vi "LDA_analogue_start_time_sync_PN.vi"(4 "Correlation peak fit method":enum32{"Max", "Quadratic", "Gaussian"}(ring)=enum."Quadratic", 5 "Pulse high threshold (Volts)":dbl=2.5, 6 "Analogue dt (s)":dbl, 7 "Analogue LDA burst pulse array":dbl[](array[numeric]), 8 "LDA arrival dt array":dbl[](array[numeric])) -> (1 "valid bursts checksum status":bool=TRUE, 2 "Absolute LDA times (s)":dbl[](array[numeric]), 3 "LDA start time rel. to Analogue (s)":dbl)   [LabVIEW 2010]
uses:
  <vilib>/Analysis/2dsp.llb/1D Cross Correlation (DBL).vi
  <vilib>/Analysis/1siggen.llb/Ramp Pattern by Samples.vi
  <vilib>/analysis/polynomials.llb/nth Derivative of Polynomial (DBL).vi
  <vilib>/analysis/polynomials.llb/Polynomial Roots (DBL).vi
  <vilib>/Analysis/NI_AALPro.lvlib
  <vilib>/Analysis/NI_AALBase.lvlib
panel:
  out "Xcorr LDA timings":cluster{"Ramp Pattern":dbl[], dbl[]}[](graph)
  in  "Pts. either side of peak to use in fit":i32=3
  out "Analogue LDA burst pulse array":cluster{"index (row)":dbl, dbl, "Vout":dbl[]}(graph)
  out "Thresholded LDA burst times (valid only)":cluster{"index (row)":dbl, dbl, "Vout":dbl[]}(graph)
  out "Thresholded LDA arr time checksum":i32
  out "Thresholded LDA burst times (valid + invalid)":cluster{"index (row)":dbl, dbl, "Vout":dbl[]}(graph)
  out "LDA counted pulses (valid + invalid)":i32
  out "LDA arr_t length":i32
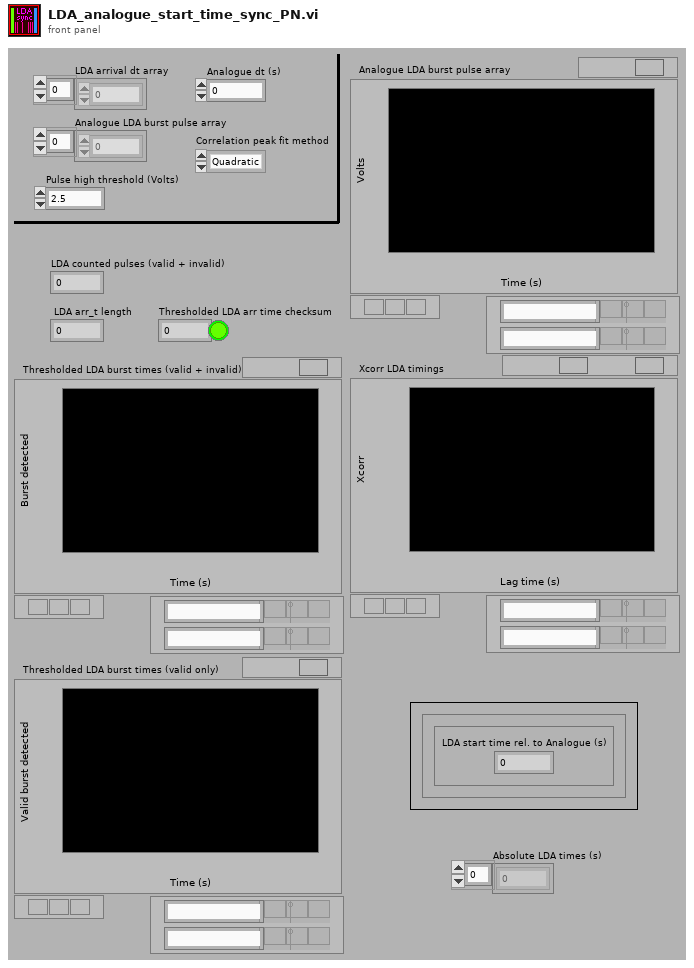
[diagram p1: front panel]
types:
  T1 = cluster{"index (row)":dbl, "Analogue dt (s)":dbl, "Vout":dbl[]}
  T2 = cluster{"index (row)":dbl, "Analogue dt (s)":dbl, "Analogue LDA burst pulse array":dbl[]}
  T3 = cluster{"Ramp Pattern":dbl[], "Best Gaussian Fit":dbl[]}[]
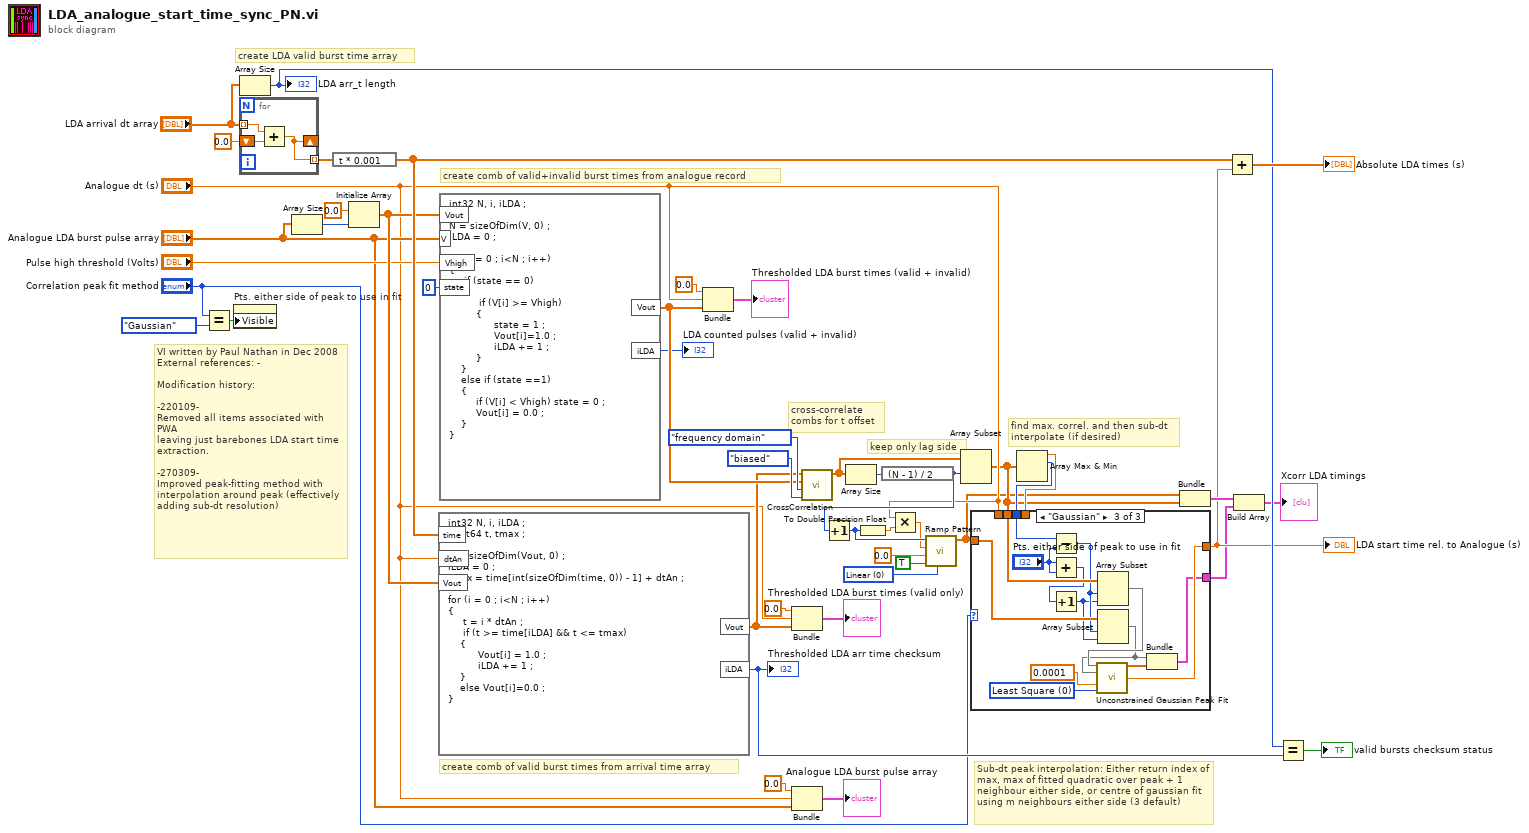
[diagram p0: block diagram]
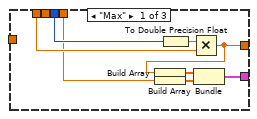
[diagram p2: hidden frame]
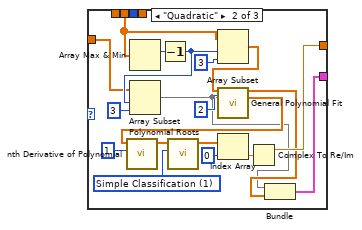
[diagram p3: hidden frame]
diagram:
  w10 = u16 0 items=["Linear", "Logarithmic"] ("type")
  # "find max. correl. and then sub-dt interpolate (if desired)"
  # "Sub-dt peak interpolation: Either return index of max, max of fitted quadratic over peak + 1 neighbour either side, or centre of gaussian fit using m neighbours either side (3 default)"
  # "create LDA valid burst time array"
  # "keep only lag side"
  # "cross-correlate combs for t offset"
  # "VI written by Paul Nathan in Dec 2008\nExternal references: -\n\nModification history:\n\n-220109-\nRemoved all items associated with PWA\nleaving just barebones LDA start time\nextraction.\n\n-270309-\nImproved peak-fitting method with interpolation around peak (effectively adding sub-dt resolution)"
  # "create comb of valid+invalid burst times from analogue record"
  # "create comb of valid burst times from arrival time array"
  n1 = Equal?(x="Correlation peak fit method", y=enum32{"Max", "Quadratic", "Gaussian"}."Gaussian") -> (x = y?=w2:bool)
  n2 = property on="Pts. either side of peak to use in fit" class="DigNum (strict)"("Visible"=w2) -> ()  [unwired: 2 in, 2 out]
  n3 = Array Size(array="LDA arrival dt array") -> (size(s)=w26:i32)
  "LDA arr_t length" <- w26
  n4 = for {
    tunnel: "LDA arrival dt array" -> [w49] mode=indexing
    shift-right: [w47] -> _
    shift-left: 0.0 ("input variable") -> [w48]
    tunnel: [w47] -> w44 mode=indexing
    n5 = Add(x=w49, y=w48) -> (x+y=w47:dbl)
  }
  n6 = Array Size(array="Analogue LDA burst pulse array") -> (size(s)=w31:i32)
  n7 = expression code="t * 0.001"(w44) -> (w32:dbl[])
  n8 = Initialize Array(0.0 ("element"), w31) -> (w30:dbl[])
  n9 = formula code="int32 N, i, iLDA ;\nfloat64 t, tmax ;\n\nN = sizeOfDim(Vout, 0) ;\niLDA = 0 ;\ntmax = time[int(sizeOfDim(time, 0)) - 1] + dtAn ;\n\nfor (i = 0 ; i<N ; i++)\n{\n     t = i * dtAn ;\n     if (t >= time[iLDA] && t <= tmax) \n    {\n          Vout[i] = 1.0 ;\n          iLDA += 1 ;\n    }\n    else Vout[i]=0.0 ;\n}"("dtAn"="Analogue dt (s)", "time"=w32, "Vout"=w30) -> ("Vout"=w35:dbl[], "iLDA"=w29:i32)
  "Thresholded LDA arr time checksum" <- w29
  n10 = formula code="int32 N, i, iLDA ;\n\nN = sizeOfDim(V, 0) ;\niLDA = 0 ;\n\nfor (i = 0 ; i<N ; i++)\n{\n     if (state == 0) \n    {\n          if (V[i] >= Vhigh)\n         {\n               state = 1 ;\n               Vout[i]=1.0 ;\n               iLDA += 1 ;\n         }\n    }\n    else if (state ==1)\n    {\n         if (V[i] < Vhigh) state = 0 ;\n         Vout[i] = 0.0 ;\n    }\n}"("V"="Analogue LDA burst pulse array", "Vhigh"="Pulse high threshold (Volts)", "state"=u8 0 ("input variable"), "Vout"=w30) -> ("Vout"=w36:dbl[], "iLDA"=→"LDA counted pulses (valid + invalid)":i32)
  n11 = Bundle("index (row)"=0.0, "Analogue dt (s)"="Analogue dt (s)", "Vout"=w36) -> (→"Thresholded LDA burst times (valid + invalid)":T1)  [unwired: 1 out]
  n12 = Bundle("index (row)"=0.0, "Analogue dt (s)"="Analogue dt (s)", "Vout"=w35) -> (→"Thresholded LDA burst times (valid only)":T1)  [unwired: 1 out]
  n13 = Bundle("index (row)"=0.0, "Analogue dt (s)"="Analogue dt (s)", "Analogue LDA burst pulse array"="Analogue LDA burst pulse array") -> (→"Analogue LDA burst pulse array":T2)  [unwired: 1 out]
  n14 = call-poly <vilib>:"CrossCorrelation.vi"("normalization"=enum32{"none", "unbiased", "biased"}."biased", "algorithm"=enum32{"direct", "frequency domain"}."frequency domain", "Y"=w36, "X"=w35) -> ("Rxy"=w33:dbl[])  [unwired: 7 out]
  n15 = Array Size(array=w33) -> (size(s)=w34:i32)
  n16 = expression code="(N - 1) / 2"(w34) -> (w12:i32)
  n17 = Increment(x=w12) -> (x+1=w19:i32)
  n18 = To Double Precision Float(number=w19) -> (double precision float=w17:dbl)
  n19 = Multiply(x="Analogue dt (s)", y=w17) -> (x*y=w18:dbl)
  n20 = call-poly <vilib>:"Ramp Pattern.vi"("type"=w10, "exclude end?"=TRUE, "start"=0.0, "end"=w18, "samples"=w19) -> ("Ramp Pattern"=w5:dbl[])  [unwired: 5 in, 1 out]
  n21 = Array Subset(array=w33, index=w12) -> (w6:dbl[])  [unwired: 1 in]
  n22 = Array Max & Min(array=w6) -> (max value=w8:dbl, max index (indices)=w9:i32)  [unwired: 2 out]
  n23 = case shown="\"Gaussian\"" "Correlation peak fit method" {
    tunnel: w6 -> [_ w65 w87]
    tunnel: [w50 w66 w89] -> w7
    tunnel: "Analogue dt (s)" -> [w57 _ _]
    tunnel: [w54 w63 w79] -> w4
    tunnel: w5 -> [_ w59 w84]
    tunnel: w9 -> [w55 _ w86]
    tunnel: w8 -> [w51 _ _]
    frame "Max" {
      n24 = Build Array(w51) -> (w53:dbl[])
      n25 = To Double Precision Float(number=w55) -> (double precision float=w56:dbl)
      n26 = Multiply(x=w56, y=w57) -> (x*y=w50:dbl)
      n27 = Build Array(w50) -> (w52:dbl[])
      n28 = Bundle(w52, w53) -> (w54:cluster{dbl[], dbl[]})  [unwired: 1 out]
    }
    frame "Quadratic" {
      w70 = u16 1 items=["General", "Simple Classification", "Refinement", "Advanced Refinement"] ("option")
      n29 = Array Max & Min(array=w65) -> (max index (indices)=w75:i32)  [unwired: 3 out]
      n30 = Decrement(x=w75) -> (x-1=w60:i32)
      n31 = Array Subset(array=w59, index=w60, length=3) -> (w58:dbl[])
      n32 = Array Subset(array=w65, index=w60, length=3) -> (w74:dbl[])
      n33 = call <vilib>:"General Polynomial Fit.vi"("Y"=w74, "polynomial order"=2, "X"=w58) -> ("Best Polynomial Fit"=w62:dbl[], "Polynomial Coefficients"=w64:dbl[])  [unwired: 9 in, 2 out]
      n34 = call-poly <vilib>:"nth Derivative of Polynomial.vi"("order"=1, "P(x)"=w64) -> ("Nth Derivative of P(x)"=w71:dbl[])  [unwired: 9 out]
      n35 = call-poly <vilib>:"Polynomial Roots.vi"("option"=w70, "P(x)"=w71) -> ("Roots"=w69:cdb[])  [unwired: 9 out]
      n36 = Index Array(array=w69, index=0) -> (element=w67:cdb)
      n37 = Complex To Re/Im(x + iy=w67) -> (x=w66:dbl)  [unwired: 1 out]
      n38 = Bundle(w58, "Best Polynomial Fit"=w62) -> (w63:cluster{dbl[], "Best Polynomial Fit":dbl[]})  [unwired: 1 out]
    }
    frame "Gaussian" {
      w88 = u16 0 items=["Least Square", "Least Absolute Residual", "Bisquare"] ("method")
      n39 = Subtract(x=w86, y="Pts. either side of peak to use in fit") -> (x-y=w83:i32)
      n40 = Add(x="Pts. either side of peak to use in fit", y="Pts. either side of peak to use in fit") -> (x+y=w77:i32)
      n41 = Increment(x=w77) -> (x+1=w78:i32)
      n42 = Array Subset(array=w87, index=w83, length=w78) -> (w82:dbl[])
      n43 = Array Subset(array=w84, index=w83, length=w78) -> (w80:dbl[])
      n44 = call <vilib>:"Unconstrained Gaussian Peak Fit.vi"("Y"=w82, "X"=w80, "tolerance"=0.0001, "method"=w88) -> ("Best Gaussian Fit"=w81:dbl[], "center"=w89:dbl)  [unwired: 6 in, 4 out]
      n45 = Bundle(w80, "Best Gaussian Fit"=w81) -> (w79:cluster{dbl[], "Best Gaussian Fit":dbl[]})  [unwired: 1 out]
    }
  }
  "LDA start time rel. to Analogue (s)" <- w7
  n46 = Bundle("Ramp Pattern"=w5, w6) -> (w13:cluster{"Ramp Pattern":dbl[], dbl[]})  [unwired: 1 out]
  n47 = Add(x=w32, y=w7) -> (x+y=→"Absolute LDA times (s)":dbl[])
  n48 = Build Array(w13, w4) -> (→"Xcorr LDA timings":T3)
  n49 = Equal?(x=w26, y=w29) -> (x = y?=→"valid bursts checksum status":bool)
